vi "Play Preview.vi"(8 "error in (no error)":errorcluster, 11 "stop":bool) -> (0 "Error Out":errorcluster, 3 "Preview":picture)   [LabVIEW 2022 SP3]
doc: "This example VI demonstrates how to acquire and display the preview image from a Phantom Camera using the Vision Research Phantom Series LabVIEW Driver. Also demonstrated is the creation of an image histogram."
uses:
  <instrlib>/Vision Research Phantom Series Labview Driver/_Type Defs/PhInt PhProcessImage Selectors.ctl
  <instrlib>/Vision Research Phantom Series Labview Driver/_Type Defs/PhInt REDUCE16TO8PARAMS.ctl
  <instrlib>/Vision Research Phantom Series Labview Driver/_Type Defs/PHCon IMRANGE.ctl
  <instrlib>/Vision Research Phantom Series Labview Driver/_Type Defs/PhFile InfName.ctl
  <instrlib>/Vision Research Phantom Series Labview Driver/VRI.lvlib
panel:
  in  "REDUCE16TO8PARAMS":T1={"fGain16_8"=1.0}
  in  "procID":T2=1 items=["IMG_PROC_REDUCE16TO8"=1]
  in  "Camera Number":u32
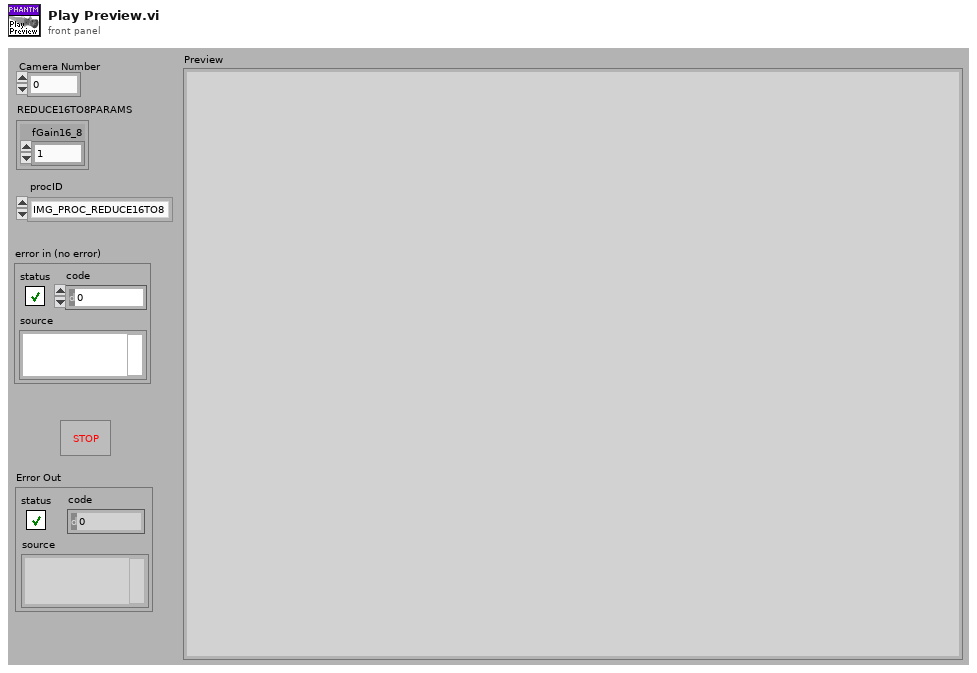
[diagram p1: front panel]
types:
  T1 = typedef "VRI.lvlib/PhInt REDUCE16TO8PARAMS.ctl" = cluster{"fGain16_8":dbl}
  T2 = typedef "VRI.lvlib/PhInt PhProcessImage Selectors.ctl" = u16
  T3 = typedef "VRI.lvlib/PhFile InfName.ctl" = u32
  T4 = typedef "VRI.lvlib/PHCon IMRANGE.ctl" = cluster{"First":i32, "Cnt":u32}
  T5 = typedef "VRI.lvlib/PhInt IH.ctl" = cluster{"biSize":u32, "biWidth":i32, "biHeight":i32, "biPlanes":u16, "biBitCount":u16, "biCompresssion":u32, "biSizeImage":u32, "biXPelsPerMeter":i32, "biYPelsPerMeter":i32, "biClrUsed":u32, "biClrImportant":u32, "BlackLevel":i32, "WhiteLevel":i32}
  T6 = typedef "VRI.lvlib/BITMAPINFOHEADER.ctl" = cluster{"biSize":u32, "biWidth":i32, "biHeight":i32, "biPlanes":u16, "biBitCount":u16, "biCompression":u32, "biSizeImage":u32, "biXPelsPerMeter":i32, "biYPelsPerMeter":i32, "biClrUsed":u32, "biClrImportant":u32}
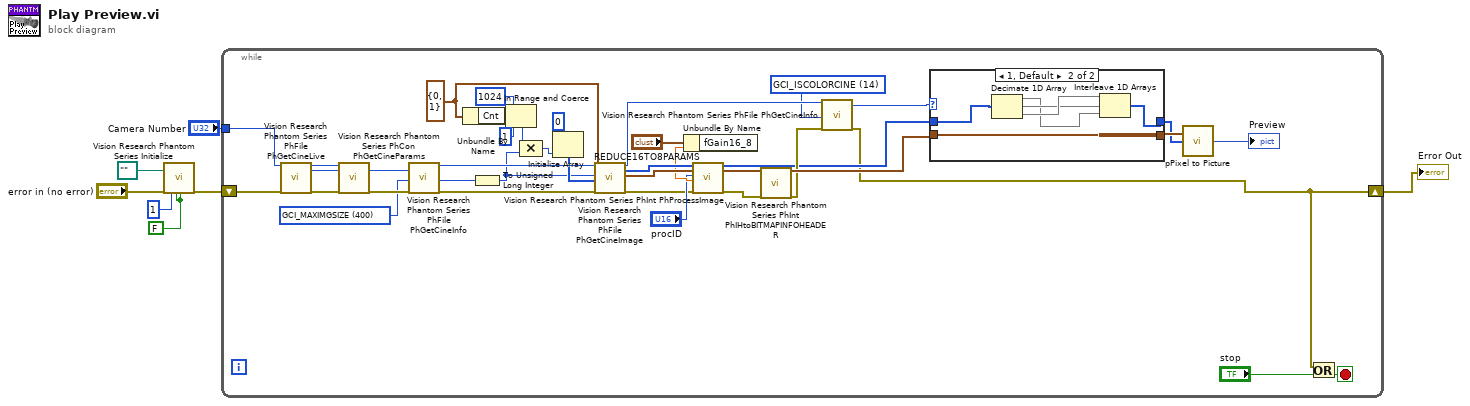
[diagram p0: block diagram]
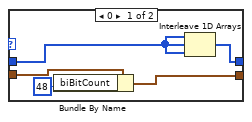
[diagram p2: hidden frame]
diagram:
  w4 = FALSE ("ID Query (T: Check)")
  n1 = call <instrlib>:"Vision Research Phantom Series Initialize.vi"("Storage Path (\"\")"=path "" ("Storage Path (\"\")"), "error in (no error)"="error in (no error)", "CallID"=u32 1, "ID Query (T: Check)"=w4, "Reset (F: Don't Reset)"=w4) -> ("Error Out"=w2:errorcluster)  [unwired: 14 out]
  n2 = while {
    tunnel: "Camera Number" -> [w22]
    shift-right: [w8] -> w1
    shift-left: w2 -> [w20]
    stop <- w9 stop-if-true
    w10 = T3 14 items=["GCI_CFA"=0, "GCI_FRAMERATE"=1, "GCI_EXPOSURE"=2, "GCI_AUTOEXPOSURE"=3, "GCI_REALBPP"=4, "GCI_CAMERASERIAL"=5, "GCI_HEADSERIAL0"=6, "GCI_HEADSERIAL1"=7, "GCI_HEADSERIAL2"=8, "GCI_HEADSERIAL3"=9, "GCI_TRIGTIMESEC"=10, "GCI_TRIGTIMEFR"=11, "GCI_ISFILECINE"=12, "GCI_IS16BPPCINE"=13, "GCI_ISCOLORCINE"=14, "GCI_ISMULTIHEADCINE"=15, "GCI_EXPOSURENS"=16, "GCI_EDREXPOSURENS"=17, "GCI_FRAMEDELAYNS"=19, "GCI_FROMFILETYPE"=20, "GCI_COMPRESSION"=21, "GCI_CAMERAVERSION"=22, "GCI_ROTATE"=23, "GCI_IMWIDTH"=24, "GCI_IMHEIGHT"=25, "GCI_IMWIDTHACQ"=26, "GCI_IMHEIGHTACQ"=27, "GCI_POSTTRIGGER"=28, "GCI_IMAGECOUNT"=29, "GCI_TOTALIMAGECOUNT"=30, "GCI_TRIGFRAME"=31, "GCI_AUTOEXPLEVEL"=32, "GCI_AUTOEXPTOP"=33, "GCI_AUTOEXPLEFT"=34, "GCI_AUTOEXPBOTTOM"=35, "GCI_AUTOEXPRIGHT"=36, "GCI_RECORDINGTIMEZONE"=37, "GCI_FIRSTIMAGENO"=38, "GCI_FIRSTMOVIEIMAGE"=39, "GCI_CINENAME"=40, "GCI_FRPSTEPS"=100, "GCI_FRP1X"=101, "GCI_FRP1Y"=102, "GCI_FRP2X"=103, "GCI_FRP2Y"=104, "GCI_FRP3X"=105, "GCI_FRP3Y"=106, "GCI_FRP4X"=107, "GCI_FRP4Y"=108, "GCI_WRITEERR"=109, "GCI_LENSDESCRIPTION"=110, "GCI_LENSAPERATURE"=111, "GCI_LENSFOCALLENGTH"=112, "GCI_WB"=200, "GCI_WBVIEW"=201, "GCI_BRIGHT"=202, "GCI_CONTRAST"=203, "GCI_GAMMA"=204, "GCI_GAMMAR"=223, "GCI_GAMMAB"=224, "GCI_SATURATION"=205, "GCI_HUE"=206, "GCI_FLIPH"=207, "GCI_FLIPV"=208, "GCI_FILTERCODE"=209, "GCI_IMFILTER"=210, "GCI_INTALGO"=211, "GCI_PEDESTALR"=212, "GCI_PEDESTALG"=213, "GCI_PEDESTALB"=214, "GCI_FLARE"=225, "GCI_CHROMA"=226, "GCI_TONE"=227, "GCI_ENABLEMATRICES"=228, "GCI_USERMATRIX"=229, "GCI_RESAMPLEACTIVE"=215, "GCI_RESAMPLEWIDTH"=216, "GCI_RESAMPLEHEIGHT"=217, "GCI_CROPACTIVE"=218, "GCI_CROPRECTANGLE"=219, "GCI_OFFSET16_8"=220, "GCI_GAIN16_8"=221, "GCI_DEMOSAICINGFUNCPTR"=222, "GCI_VFLIPVIEWACTIVE"=300, "GCI_MAXIMGSIZE"=400, "GCI_FRPIMGNOARRAY"=450, "GCI_FRPRATEARRAY"=451, "GCI_FRPSHAPEARRAY"=452, "GCI_TRIGTC"=470, "GCI_TRIGTCU"=471, "GCI_PBRATE"=472, "GCI_TCRATE"=473, "GCI_SAVERANGE"=500, "GCI_SAVEFILENAME"=501, "GCI_SAVEFILETYPE"=502, "GCI_SAVE16BIT"=503, "GCI_SAVEPACKED"=504, "GCI_SAVEXML"=505, "GCI_SAVESTAMPTIME"=506, "GCI_SAVEAVIFRAMERATE"=520, "GCI_SAVEAVICOMPRESSORLIST"=521, "GCI_SAVEAVICOMPRESSORINDEX"=522, "GCI_SAVEDPXLSB"=530, "GCI_SAVEDPXTO10BPS"=531, "GCI_SAVEDPXDATAPACKING"=532, "GCI_SAVEDPX10BITLOG"=533, "GCI_SAVEDPXEXPORTLOGLUT"=534, "GCI_SAVEDPX10BITLOGREFWHITE"=535, "GCI_SAVEDPX10BITLOGREFBLACK"=536, "GCI_SAVEDPX10BITLOGGAMMA"=537, "GCI_SAVEDPX10BITLOGFILMGAMMA"=538, "GCI_SAVEQTPLAYBACKRATE"=550, "GCI_SAVECCIQUALITY"=560, "GCI_UNCALIBRATEDIMAGE"=600, "GCI_NOPROCESSING"=601, "GCI_BADPIXELREPAIR"=602] ("InfName")
    w21 = T3 400 items=["GCI_CFA"=0, "GCI_FRAMERATE"=1, "GCI_EXPOSURE"=2, "GCI_AUTOEXPOSURE"=3, "GCI_REALBPP"=4, "GCI_CAMERASERIAL"=5, "GCI_HEADSERIAL0"=6, "GCI_HEADSERIAL1"=7, "GCI_HEADSERIAL2"=8, "GCI_HEADSERIAL3"=9, "GCI_TRIGTIMESEC"=10, "GCI_TRIGTIMEFR"=11, "GCI_ISFILECINE"=12, "GCI_IS16BPPCINE"=13, "GCI_ISCOLORCINE"=14, "GCI_ISMULTIHEADCINE"=15, "GCI_EXPOSURENS"=16, "GCI_EDREXPOSURENS"=17, "GCI_FRAMEDELAYNS"=19, "GCI_FROMFILETYPE"=20, "GCI_COMPRESSION"=21, "GCI_CAMERAVERSION"=22, "GCI_ROTATE"=23, "GCI_IMWIDTH"=24, "GCI_IMHEIGHT"=25, "GCI_IMWIDTHACQ"=26, "GCI_IMHEIGHTACQ"=27, "GCI_POSTTRIGGER"=28, "GCI_IMAGECOUNT"=29, "GCI_TOTALIMAGECOUNT"=30, "GCI_TRIGFRAME"=31, "GCI_AUTOEXPLEVEL"=32, "GCI_AUTOEXPTOP"=33, "GCI_AUTOEXPLEFT"=34, "GCI_AUTOEXPBOTTOM"=35, "GCI_AUTOEXPRIGHT"=36, "GCI_RECORDINGTIMEZONE"=37, "GCI_FIRSTIMAGENO"=38, "GCI_FIRSTMOVIEIMAGE"=39, "GCI_CINENAME"=40, "GCI_FRPSTEPS"=100, "GCI_FRP1X"=101, "GCI_FRP1Y"=102, "GCI_FRP2X"=103, "GCI_FRP2Y"=104, "GCI_FRP3X"=105, "GCI_FRP3Y"=106, "GCI_FRP4X"=107, "GCI_FRP4Y"=108, "GCI_WRITEERR"=109, "GCI_LENSDESCRIPTION"=110, "GCI_LENSAPERATURE"=111, "GCI_LENSFOCALLENGTH"=112, "GCI_WB"=200, "GCI_WBVIEW"=201, "GCI_BRIGHT"=202, "GCI_CONTRAST"=203, "GCI_GAMMA"=204, "GCI_GAMMAR"=223, "GCI_GAMMAB"=224, "GCI_SATURATION"=205, "GCI_HUE"=206, "GCI_FLIPH"=207, "GCI_FLIPV"=208, "GCI_FILTERCODE"=209, "GCI_IMFILTER"=210, "GCI_INTALGO"=211, "GCI_PEDESTALR"=212, "GCI_PEDESTALG"=213, "GCI_PEDESTALB"=214, "GCI_FLARE"=225, "GCI_CHROMA"=226, "GCI_TONE"=227, "GCI_ENABLEMATRICES"=228, "GCI_USERMATRIX"=229, "GCI_RESAMPLEACTIVE"=215, "GCI_RESAMPLEWIDTH"=216, "GCI_RESAMPLEHEIGHT"=217, "GCI_CROPACTIVE"=218, "GCI_CROPRECTANGLE"=219, "GCI_OFFSET16_8"=220, "GCI_GAIN16_8"=221, "GCI_DEMOSAICINGFUNCPTR"=222, "GCI_VFLIPVIEWACTIVE"=300, "GCI_MAXIMGSIZE"=400, "GCI_FRPIMGNOARRAY"=450, "GCI_FRPRATEARRAY"=451, "GCI_FRPSHAPEARRAY"=452, "GCI_TRIGTC"=470, "GCI_TRIGTCU"=471, "GCI_PBRATE"=472, "GCI_TCRATE"=473, "GCI_SAVERANGE"=500, "GCI_SAVEFILENAME"=501, "GCI_SAVEFILETYPE"=502, "GCI_SAVE16BIT"=503, "GCI_SAVEPACKED"=504, "GCI_SAVEXML"=505, "GCI_SAVESTAMPTIME"=506, "GCI_SAVEAVIFRAMERATE"=520, "GCI_SAVEAVICOMPRESSORLIST"=521, "GCI_SAVEAVICOMPRESSORINDEX"=522, "GCI_SAVEDPXLSB"=530, "GCI_SAVEDPXTO10BPS"=531, "GCI_SAVEDPXDATAPACKING"=532, "GCI_SAVEDPX10BITLOG"=533, "GCI_SAVEDPXEXPORTLOGLUT"=534, "GCI_SAVEDPX10BITLOGREFWHITE"=535, "GCI_SAVEDPX10BITLOGREFBLACK"=536, "GCI_SAVEDPX10BITLOGGAMMA"=537, "GCI_SAVEDPX10BITLOGFILMGAMMA"=538, "GCI_SAVEQTPLAYBACKRATE"=550, "GCI_SAVECCIQUALITY"=560, "GCI_UNCALIBRATEDIMAGE"=600, "GCI_NOPROCESSING"=601, "GCI_BADPIXELREPAIR"=602] ("InfName")
    w23 = T4 {"First"=0, "Cnt"=1} ("pRng")
    n3 = call <instrlib>:"Vision Research Phantom Series PhFile PhGetCineLive.vi"("CN (in)"=w22, "Error In (no error)"=w20) -> ("CN (out)"=w29:u32, "pCH (out)"=w43:u64, "Error Out"=w31:errorcluster)  [unwired: 15 in]
    n4 = call <instrlib>:"Vision Research Phantom Series PhCon PhGetCineParams.vi"("CN in"=w29, "Error In (no error)"=w31) -> ("Error Out"=w30:errorcluster)  [unwired: 1 in, 16 out]
    n5 = call <instrlib>:"Vision Research Phantom Series PhFile PhGetCineInfo.vi"("CH in"=w43, "InfName"=w21, "Error In (no error)"=w30) -> ("CH out"=w41:u64, "pInfVal out"=w14:i32, "Error Out"=w39:errorcluster)  [unwired: 14 in]
    n6 = Unbundle By Name(w23) -> ("Cnt"=w28:u32)
    n7 = To Unsigned Long Integer(number=w14) -> (unsigned 32bit integer=w13:u32)
    n8 = In Range and Coerce(upper limit=u32 1024, x=w28, lower limit=u32 1) -> (coerced(x)=w27:u32)  [unwired: 1 out]
    n9 = Compound Arithmetic op=MULTIPLY(w27, w13) -> (w24:u32)
    n10 = Initialize Array(u16 0 ("element"), w24) -> (w40:u16[])
    n11 = call <instrlib>:"Vision Research Phantom Series PhFile PhGetCineImage.vi"("hC [in]"=w41, "pRng [in]"=w23, "bufferByteSize [in]"=w13, "pPixelBuffer [in]"=w40, "Error In (no error)"=w39) -> ("hC [out]"=w19:u64, "pPixelBuffer [out]"=w38:u16[], "IH [out]"=w37:T5, "Error Out"=w34:errorcluster)  [unwired: 11 in]
    n12 = Unbundle By Name("REDUCE16TO8PARAMS") -> ("fGain16_8"=w36:dbl)
    n13 = call <instrlib>:"Vision Research Phantom Series PhInt PhProcessImage.vi"("pPixelSrc [in]"=w38, "IH [in]"=w37, "procID"="procID", "pProcParams"=w36, "Error In (no error)"=w34) -> ("pPixelDest [out]"=w11:u8[], "IH [out]"=w32:T5, "Error Out"=w33:errorcluster)  [unwired: 12 in]
    n14 = call <instrlib>:"Vision Research Phantom Series PhInt PhIHtoBITMAPINFOHEADER.vi"("IH"=w32, "Error In (no error)"=w33) -> ("BITMAPINFOHEADER"=w17:T6, "Error Out"=w15:errorcluster)  [unwired: 16 in]
    n15 = call <instrlib>:"Vision Research Phantom Series PhFile PhGetCineInfo.vi"("CH in"=w19, "InfName"=w10, "Error In (no error)"=w15) -> ("pInfVal out"=w18:i32, "Error Out"=w8:errorcluster)  [unwired: 14 in, 1 out]
    n16 = case shown="1, Default" w18 {
      tunnel: [w48 w52] -> w12
      tunnel: w17 -> [w51 w57]
      tunnel: [w50 w57] -> w16
      tunnel: w11 -> [w47 w53]
      frame 0 {
        n17 = Bundle By Name(cluster=w51, "biBitCount"=u16 48) -> (w50:T6)
        n18 = Interleave 1D Arrays(w47, w47, w47) -> (w48:u8[])
      }
      frame 1, Default {
        n19 = Decimate 1D Array(w53) -> (w54:u8[], w55:u8[], w56:u8[])
        n20 = Interleave 1D Arrays(w56, w55, w54) -> (w52:u8[])
      }
    }
    n21 = call <instrlib>:"pPixel to Picture.vi"("pPixel"=w12, "BITMAPINFOHEADER"=w16) -> ("Preview"=→"Preview":picture)  [unwired: 1 in]
    n22 = Or(x=w8, y="stop") -> (x .or. y?=w9:bool)
  }
  "Error Out" <- w1
